vi "FTW-Tag-Core_Process.vi"(0 "FTW Actor Instance Configuration":string="{\n  \"Identity\": \"ActorName\",\n  \"InboxAddress\": \"inproc://*\",\n  \"LoggerAddress\": \"\",\n  \"My Data\": false,\n  \"Publisher URI\": \"inproc://*\",\n  \"Subscriber URIs\": \"\",\n  \"Refresh Period\": 2\n}", 11 "ErrorIn":errorcluster) -> (15 "Error":errorcluster)   [LabVIEW 2015, in "FTW-Tag-Core.lvclass"]
uses:
  FTW-Tag-Core.lvclass
  FTW-Tag-Core.lvclass/FTW-Tag-Core.ctl
  JSON/FTW-JSON-JoinMode.ctl
  Instance/FTW-ActorInstance.lvclass/FTW-ActorInstance.ctl
  JobSequencer/FTW-SEQ-Current.vi
  Message/Base/FTW-Message.lvclass
  Instance/FTW-ActorInstance.lvclass
  Message/Request/FTW-Message-IncomingRequest.lvclass
  container/FTW-Container.lvclass
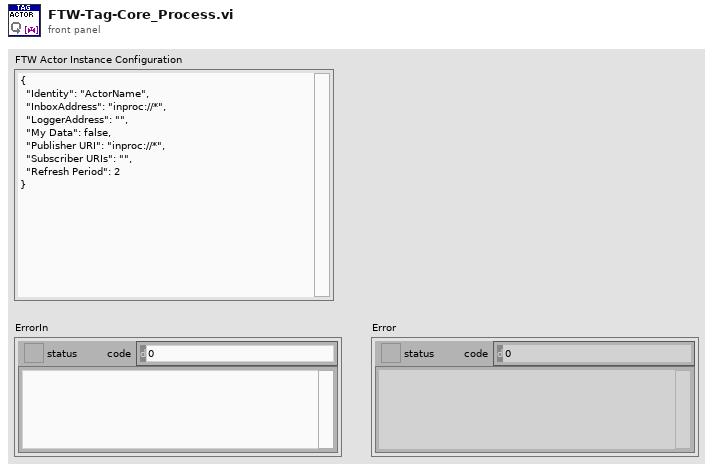
[diagram p1: front panel]
types:
  T1 = cluster{"Incoming Requests":refnum<event-registration>, "Local Messages":refnum<event-registration>, "Subscriber Registration":refnum<event-registration>}
  T2 = typedef "FTW-JSON-JoinMode.ctl" = enum32{"Upsert", "Update Only", "Insert Only"}
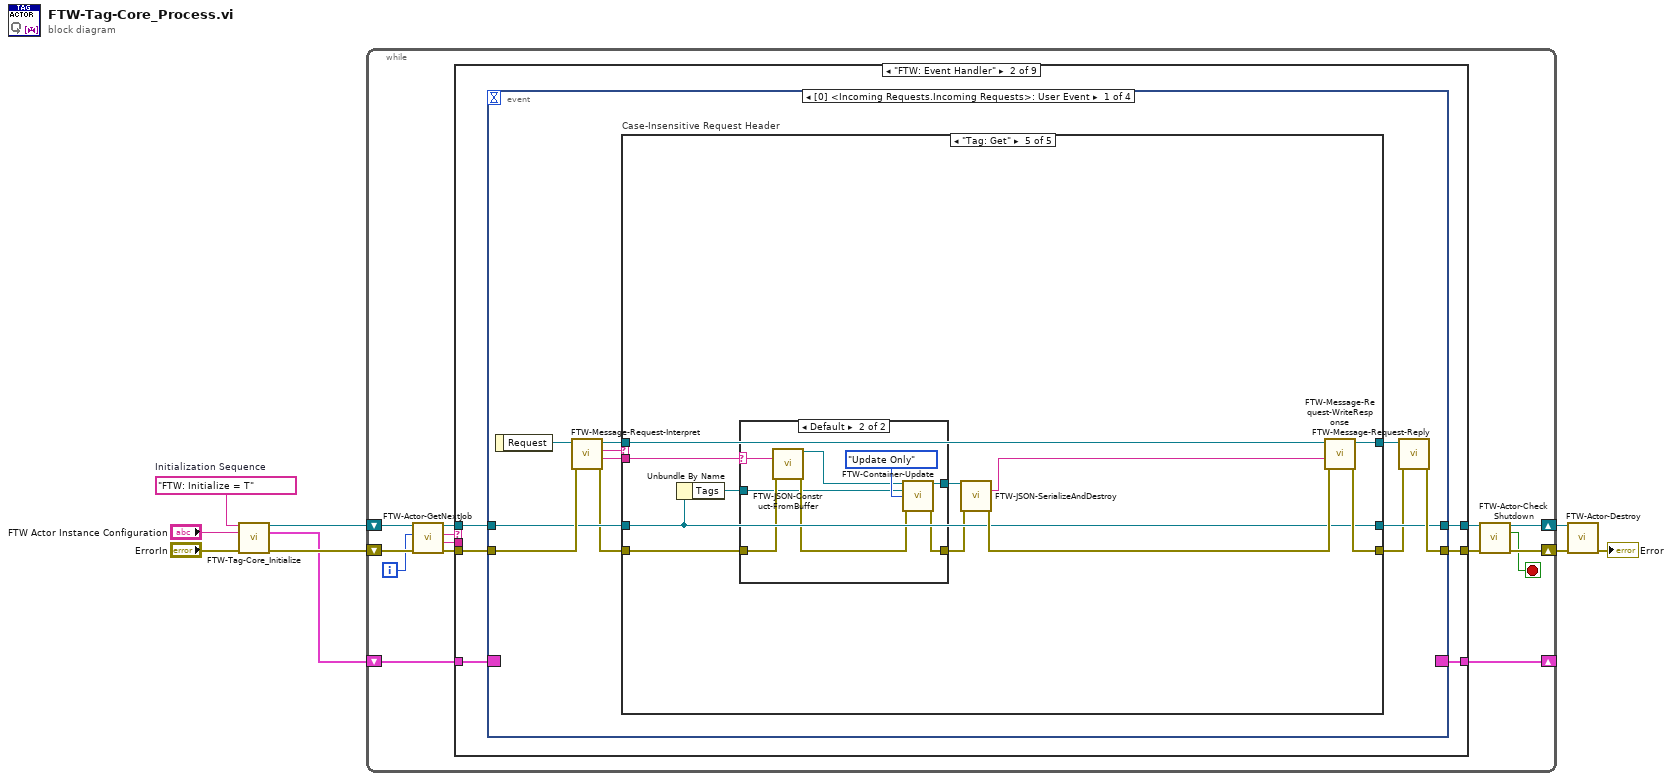
[diagram p0: block diagram]
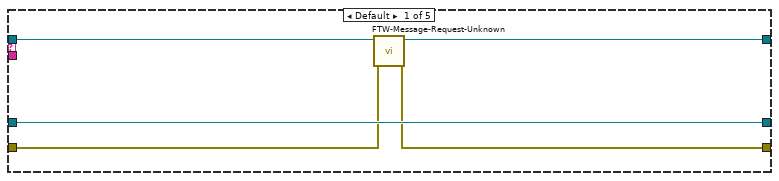
[diagram p3: hidden frame]
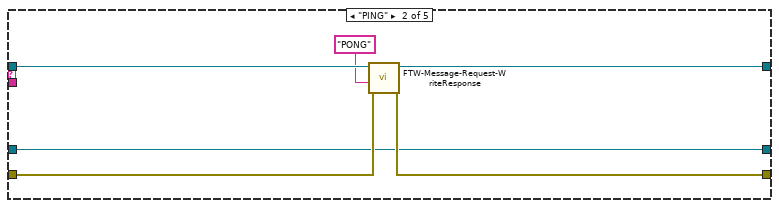
[diagram p4: hidden frame]
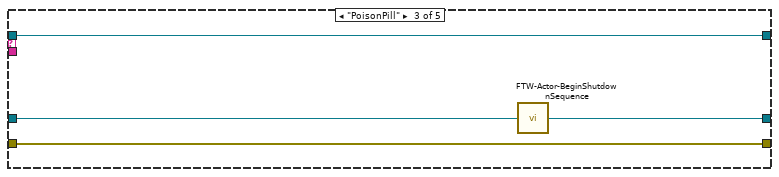
[diagram p5: hidden frame]
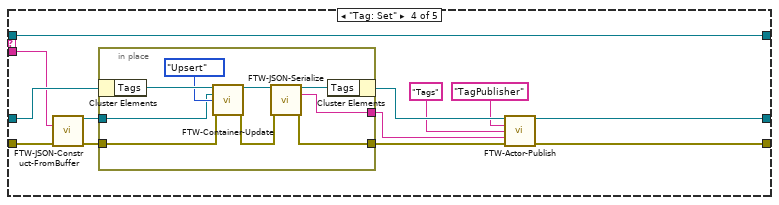
[diagram p6: hidden frame]
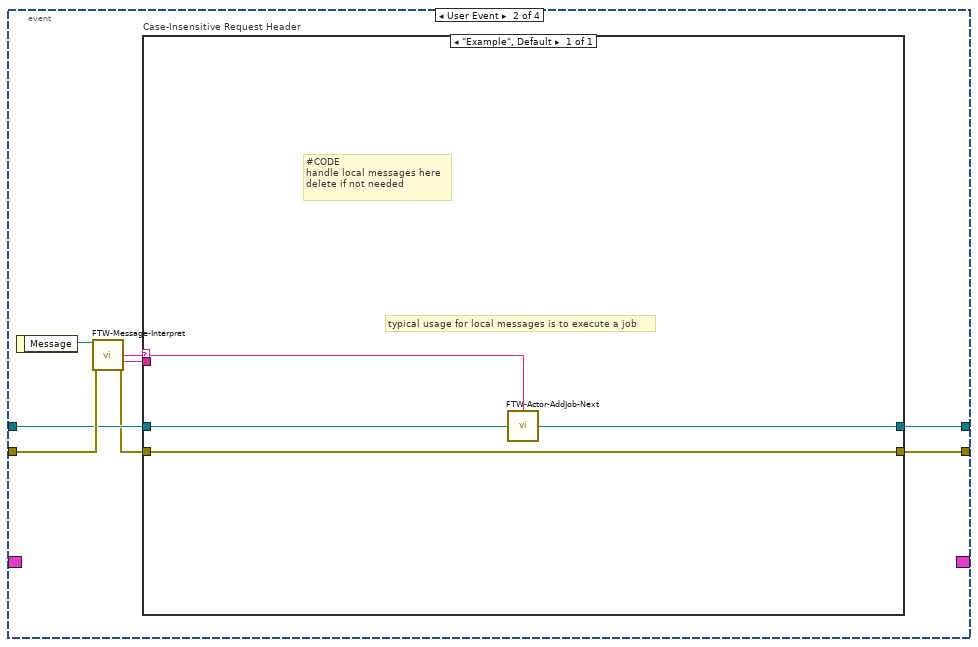
[diagram p8: hidden frame]
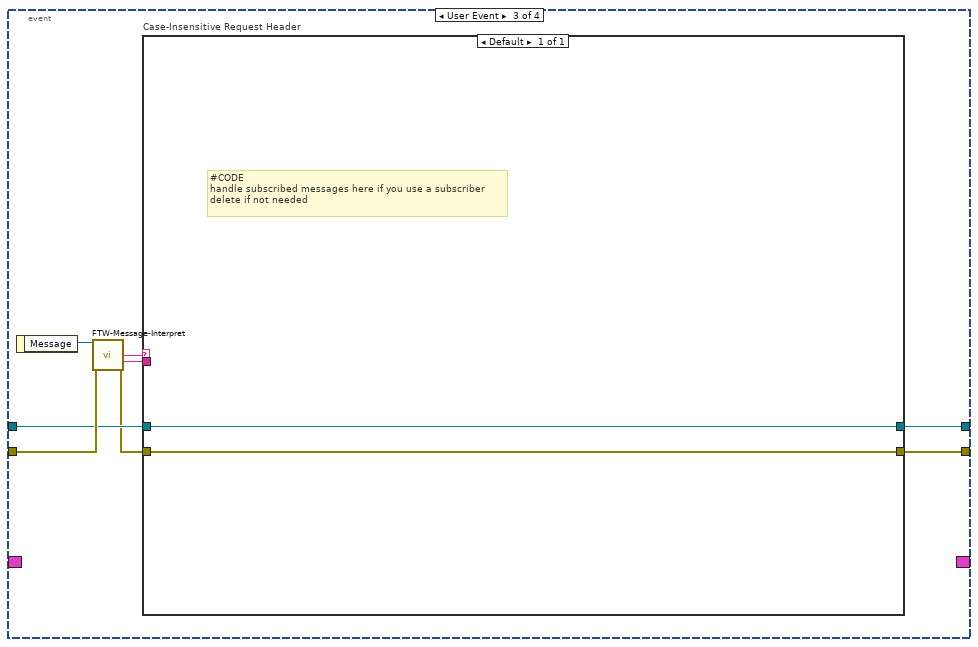
[diagram p9: hidden frame]
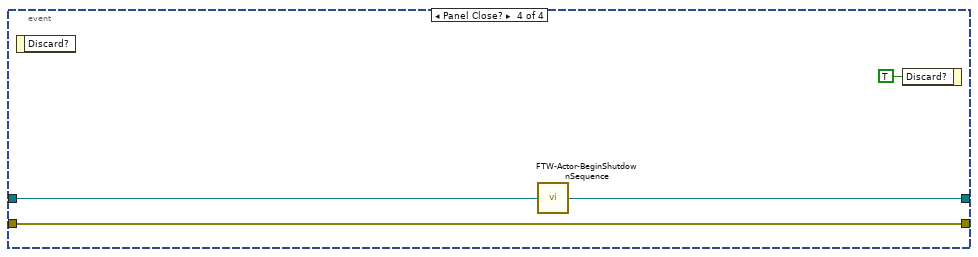
[diagram p10: hidden frame]
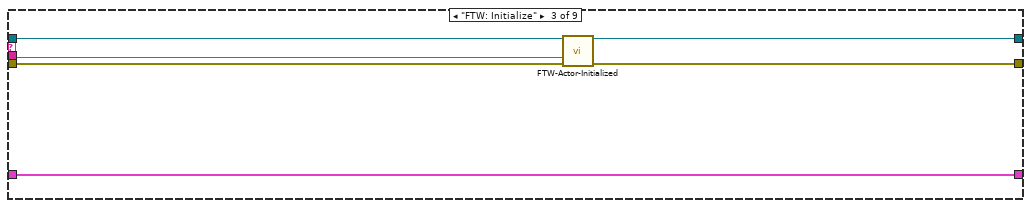
[diagram p11: hidden frame]
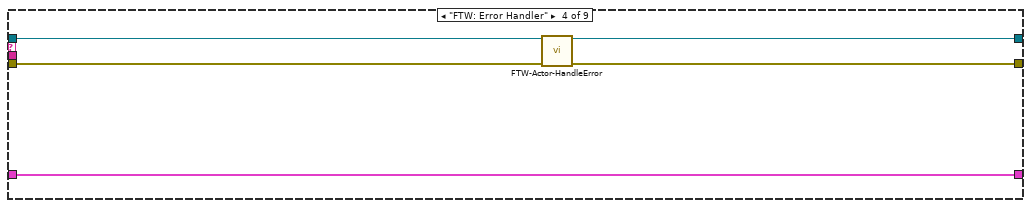
[diagram p12: hidden frame]
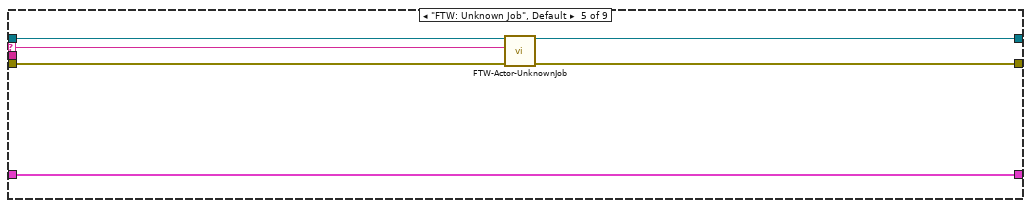
[diagram p13: hidden frame]
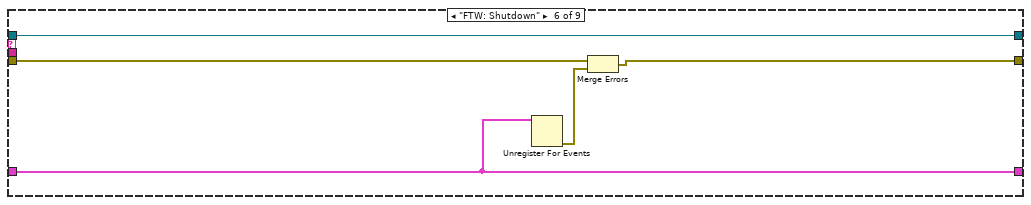
[diagram p14: hidden frame]
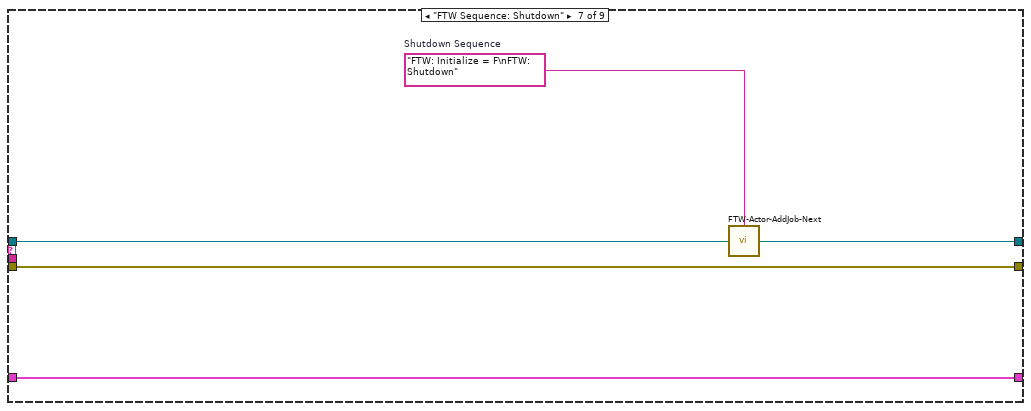
[diagram p15: hidden frame]
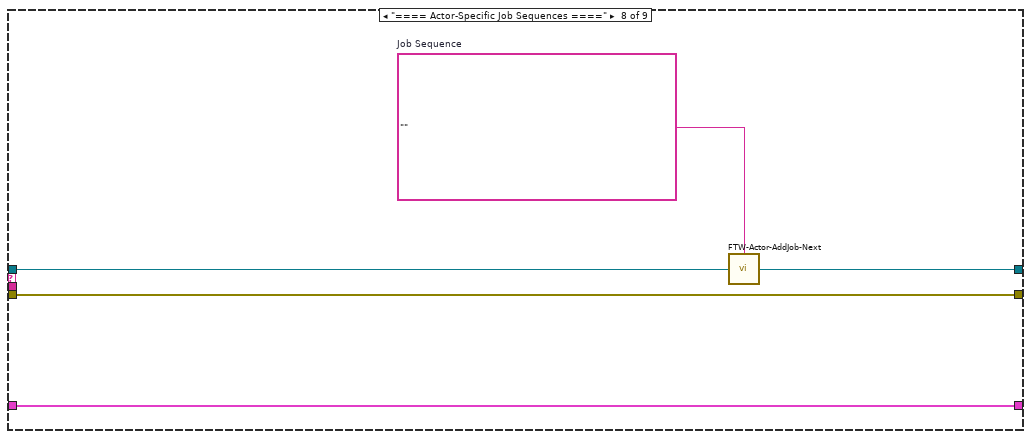
[diagram p16: hidden frame]
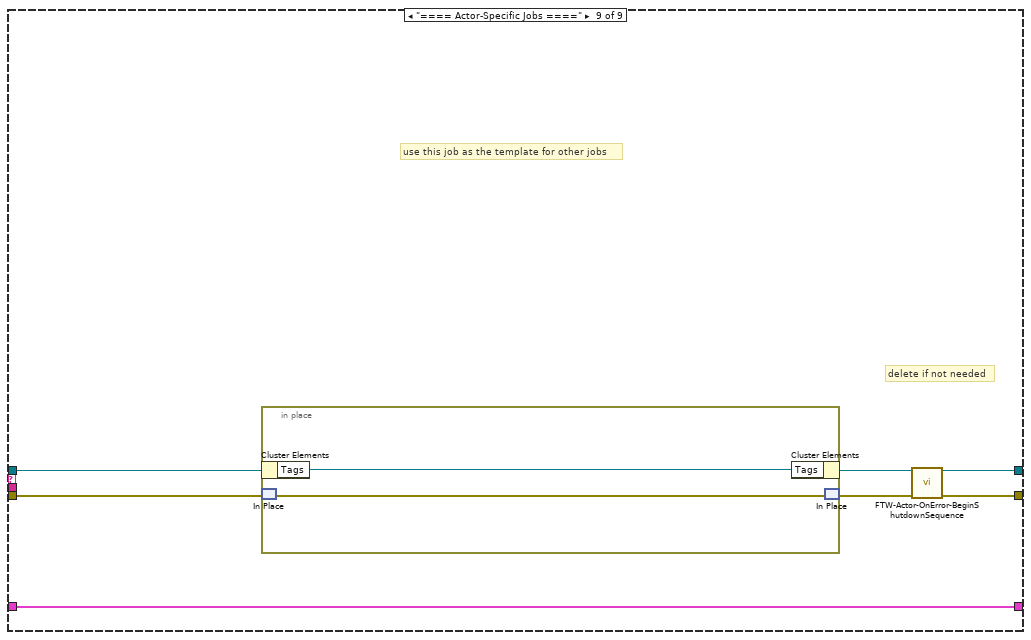
[diagram p17: hidden frame]
diagram:
  w5 = "FTW: Initialize = T"  # Initialization Sequence
  n1 = call "FTW-Tag-Core_Initialize.vi"("Initialization Sequence"=w5, "FTW Actor Instance Configuration"="FTW Actor Instance Configuration", "error in (no error)"="ErrorIn") -> ("FTW-Tag-Core Out"=w1:refnum<class "FTW-Tag-Core.lvclass">, "Event Refnums"=w2:T1, "error out"=w6:errorcluster)  [unwired: 10 in]
  n2 = while {
    shift-right: [w13] -> w8
    shift-left: w6 -> [w20]
    shift-right: [w10] -> _
    shift-left: w2 -> [w23]
    shift-right: [w15] -> w9
    shift-left: w1 -> [w22]
    i -> [w11]
    stop <- w12 stop-if-true
    n3 = call "FTW-Actor-GetNextJob.vi"("error in"=w20, "Jobs Performed"=w11, "FTW Actor Instance"=w22) -> ("error out"=w19:errorcluster, "Job Data"=w17:string, "Job Name"=w18:string, "FTW Actor Instance out"=w21:refnum<class "FTW-Tag-Core.lvclass">)  [unwired: 5 in]
    n4 = case shown="\"FTW: Event Handler\"" w18 {
      selector: w18 -> [_ _ _ _ w139 _ _ _ _]
      tunnel: [w25 w32 w130 w134 w142 w148 w153 w158 w162] -> w14
      tunnel: w19 -> [w25 w31 w133 w136 w143 w149 w153 w158 w165]
      tunnel: w23 -> [w26 w27 w132 w138 w144 w146 w154 w159 w166]
      tunnel: [w26 w30 w132 w138 w144 w146 w154 w159 w166] -> w10
      tunnel: w17 -> [_ _ w128 _ _ _ _ _ _]
      tunnel: [w24 w29 w131 w135 w140 w145 w151 w156 w160] -> w16
      tunnel: w21 -> [w24 w28 w129 w137 w141 w145 w152 w157 w163]
      frame "==== Featherweight Framework Jobs ====" {
      }
      frame "FTW: Event Handler" {
        n5 = event shown="[0] <Incoming Requests.Incoming Requests>: User Event" {
          selector: w27 -> [_ _ _ _]
          dyn-events: [_ _ _ _] -> w30
          timeout: _ -> [_ _ _ _]
          tunnel: [w42 w104 w116 w126] -> w32
          tunnel: w31 -> [w41 w108 w120 w126]
          tunnel: [w36 w105 w117 w124] -> w29
          tunnel: w28 -> [w40 w107 w119 w125]
          event User Event {
            n6 = event-data() -> ("Request"=w43:refnum<class "FTW-Message-IncomingRequest.lvclass">)  [unwired: 1 in]
            n7 = call "FTW-Message-Request-Interpret.vi"("error in"=w41, "FTW Incoming Request"=w43) -> ("error out"=w39:errorcluster, "Request Body"=w33:string, "Request Header"=w37:string, "FTW Incoming Request out"=w38:refnum<class "FTW-Message-IncomingRequest.lvclass">)  [unwired: 6 in]
            n8 = case "Case-Insensitive Request Header" shown="\"Tag: Get\"" w37 {
              tunnel: [w46 w52 w57 w64 w91] -> w35
              tunnel: w39 -> [w47 w53 w57 w70 w88]
              tunnel: [w48 w51 w58 w62 w86] -> w36
              tunnel: w40 -> [w48 w51 w56 w68 w86]
              tunnel: w38 -> [w45 w54 w55 w71 w89]
              tunnel: [w44 w50 w55 w71 w90] -> w34
              tunnel: w33 -> [_ _ _ w66 w85]
              frame Default {
                n9 = call "FTW-Message-Request-Unknown.vi"("error in"=w47, "FTW Incoming Request"=w45) -> ("error out"=w46:errorcluster, "FTW Incoming Request Out"=w44:refnum<class "FTW-Message-IncomingRequest.lvclass">)  [unwired: 8 in]
              }
              frame "PING" {
                n10 = call "FTW-Message-Request-WriteResponse.vi"("error in"=w53, "Response Body"="PONG" ("Response Header"), "FTW Incoming Request"=w54) -> ("error out"=w52:errorcluster, "FTW Incoming Request out"=w50:refnum<class "FTW-Message-IncomingRequest.lvclass">)  [unwired: 7 in]
              }
              frame "PoisonPill" {
                n11 = call "FTW-Actor-BeginShutdownSequence.vi"("FTW Actor Instance"=w56) -> ("FTW Actor Instance out"=w58:refnum<class "FTW-Tag-Core.lvclass">)  [unwired: 3 in]
              }
              frame "Tag: Set" {
                n12 = call "FTW-JSON-Construct-FromBuffer.vi"("JSON String (UTF-8)"=w66, "error in"=w70) -> ("JSON"=w65:refnum<class "FTW-Container.lvclass">, "error out"=w67:errorcluster)  [unwired: 12 in]
                n13 = in-place {
                  in-place-border: w67 -> [w80]
                  in-place-border: [w78] -> w69
                  in-place-border: [w74] -> w59
                  in-place-border: w65 -> [w72]
                  n14 = in-place-cluster #1(w68) -> ("Tags"=w76:refnum<class "FTW-Container.lvclass">)
                  n15 = call "FTW-Container-Update.vi"("FTW-Container In"=w76, "Other Container"=w72, "Join Mode"=FTW-JSON-JoinMode."Upsert", "error in"=w80) -> ("Updated Container"=w77:refnum<class "FTW-Container.lvclass">, "error out"=w79:errorcluster)  [unwired: 10 in]
                  n16 = call "FTW-JSON-Serialize.vi"("JSON"=w77, "error in"=w79) -> ("JSON out"=w75:refnum<class "FTW-Container.lvclass">, "JSON String (UTF-8)"=w74:string, "error out"=w78:errorcluster)  [unwired: 11 in]
                  n17 = in-place-cluster #1("Tags"=w75) -> (w63:refnum<class "FTW-Tag-Core.lvclass">)
                }
                n18 = call "FTW-Actor-Publish.vi"("FTW-ActorExtended In"=w63, "Publisher Name"="TagPublisher", "Message Header"="Tags", "Message Body"=w59, "error in"=w69) -> ("FTW-ActorExtended Out"=w62:refnum<class "FTW-Tag-Core.lvclass">, "error out"=w64:errorcluster)  [unwired: 9 in]
              }
              frame "Tag: Get" {
                n19 = Unbundle By Name(w86) -> ("Tags"=w81:refnum<class "FTW-Container.lvclass">)
                n20 = case shown="Default" w85 {
                  selector: w85 -> [_ w99]
                  tunnel: w88 -> [w92 w101]
                  tunnel: [w92 w98] -> w83
                  tunnel: [w93 w97] -> w82
                  tunnel: w81 -> [w93 w95]
                  frame "\u0000" {
                  }
                  frame Default {
                    n21 = call "FTW-JSON-Construct-FromBuffer.vi"("JSON String (UTF-8)"=w99, "error in"=w101) -> ("JSON"=w94:refnum<class "FTW-Container.lvclass">, "error out"=w100:errorcluster)  [unwired: 12 in]
                    n22 = call "FTW-Container-Update.vi"("FTW-Container In"=w94, "Other Container"=w95, "Join Mode"=FTW-JSON-JoinMode."Update Only", "error in"=w100) -> ("Updated Container"=w97:refnum<class "FTW-Container.lvclass">, "error out"=w98:errorcluster)  [unwired: 10 in]
                  }
                }
                n23 = call "FTW-JSON-SerializeAndDestroy.vi"("JSON"=w82, "error in"=w83) -> ("JSON String (UTF-8)"=w84:string, "error out"=w87:errorcluster)  [unwired: 12 in]
                n24 = call "FTW-Message-Request-WriteResponse.vi"("error in"=w87, "Response Body"=w84, "FTW Incoming Request"=w89) -> ("error out"=w91:errorcluster, "FTW Incoming Request out"=w90:refnum<class "FTW-Message-IncomingRequest.lvclass">)  [unwired: 7 in]
              }
            }
            n25 = call "FTW-Message-Request-Reply.vi"("FTW: Reply Error"=w35, "FTW Incoming Request"=w34) -> ("error out"=w42:errorcluster)  [unwired: 8 in, 1 out]
          }
          event User Event {
            n26 = event-data() -> ("Message"=w109:refnum<class "FTW-Message.lvclass">)  [unwired: 1 in]
            n27 = call-dynamic "FTW-Message-Interpret.vi"("FTW Message"=w109, "error in"=w108) -> ("Message Header"=w103:string, "Message Body"=w102:string, "error out"=w106:errorcluster)  [unwired: 9 in, 2 out]
            n28 = case "Case-Insensitive Request Header" shown="\"Example\", Default" w103 {
              selector: w103 -> [w110]
              tunnel: [w112] -> w104
              tunnel: w106 -> [w112]
              tunnel: [w111] -> w105
              tunnel: w107 -> [w113]
              tunnel: w102 -> [_]
              frame "Example", Default {
                # "#CODE\nhandle local messages here\ndelete if not needed"
                # "typical usage for local messages is to execute a job"
                n29 = call "FTW-Actor-AddJob-Next.vi"("Add Next in Job Queue"=w110, "FTW Actor Instance"=w113) -> ("FTW Actor Instance out"=w111:refnum<class "FTW-Tag-Core.lvclass">)  [unwired: 2 in]
              }
            }
          }
          event User Event {
            n30 = event-data() -> ("Message"=w121:refnum<class "FTW-Message.lvclass">)  [unwired: 1 in]
            n31 = call-dynamic "FTW-Message-Interpret.vi"("FTW Message"=w121, "error in"=w120) -> ("Message Header"=w115:string, "Message Body"=w114:string, "error out"=w118:errorcluster)  [unwired: 9 in, 2 out]
            n32 = case "Case-Insensitive Request Header" shown="Default" w115 {
              tunnel: [w122] -> w116
              tunnel: w118 -> [w122]
              tunnel: [w123] -> w117
              tunnel: w119 -> [w123]
              tunnel: w114 -> [_]
              frame Default {
                # "#CODE\nhandle subscribed messages here if you use a subscriber\ndelete if not needed"
              }
            }
          }
          event Panel Close? {
            n33 = event-data() -> ()  [unwired: 1 in, 1 out]
            n34 = call "FTW-Actor-BeginShutdownSequence.vi"("FTW Actor Instance"=w125) -> ("FTW Actor Instance out"=w124:refnum<class "FTW-Tag-Core.lvclass">)  [unwired: 3 in]
            n35 = event-data("Discard?"=TRUE) -> ()  [unwired: 1 in, 1 out]
          }
        }
      }
      frame "FTW: Initialize" {
        n36 = call-dynamic "FTW-Actor-Initialized.vi"("FTW Actor Instance"=w129, "Positive Init?"=w128, "error in"=w133) -> ("FTW Actor Instance out"=w131:refnum<class "FTW-Tag-Core.lvclass">, "error out"=w130:errorcluster)  [unwired: 11 in]
      }
      frame "FTW: Error Handler" {
        n37 = call-dynamic "FTW-Actor-HandleError.vi"("FTW Actor Instance"=w137, "error in"=w136) -> ("FTW Actor Instance out"=w135:refnum<class "FTW-Tag-Core.lvclass">, "error out"=w134:errorcluster)  [unwired: 10 in, 2 out]
      }
      frame "FTW: Unknown Job", Default {
        n38 = call-dynamic "FTW-Actor-UnknownJob.vi"("FTW Actor Instance"=w141, "Unknown Job"=w139, "error in"=w143) -> ("FTW Actor Instance out"=w140:refnum<class "FTW-Tag-Core.lvclass">, "error out"=w142:errorcluster)  [unwired: 11 in]
      }
      frame "FTW: Shutdown" {
        n39 = Unregister For Events(event registration refnum=w146) -> (error out=w147:errorcluster)  [unwired: 1 in]
        n40 = Merge Errors(w149, w147) -> (w148:errorcluster)
      }
      frame "FTW Sequence: Shutdown" {
        w150 = "FTW: Initialize = F\nFTW: Shutdown"  # Shutdown Sequence
        n41 = call "FTW-Actor-AddJob-Next.vi"("Add Next in Job Queue"=w150, "FTW Actor Instance"=w152) -> ("FTW Actor Instance out"=w151:refnum<class "FTW-Tag-Core.lvclass">)  [unwired: 2 in]
      }
      frame "==== Actor-Specific Job Sequences ====" {
        w155 = ""  # Job Sequence
        n42 = call "FTW-Actor-AddJob-Next.vi"("Add Next in Job Queue"=w155, "FTW Actor Instance"=w157) -> ("FTW Actor Instance out"=w156:refnum<class "FTW-Tag-Core.lvclass">)  [unwired: 2 in]
      }
      frame "==== Actor-Specific Jobs ====" {
        # "delete if not needed"
        # "use this job as the template for other jobs"
        n43 = in-place {
          n44 = in-place-cluster #2(w163) -> ("Tags"=w167:refnum<class "FTW-Container.lvclass">)
          n45 = in-place-match #3(w165) -> (w168:errorcluster)
          n46 = in-place-cluster #2("Tags"=w167) -> (w161:refnum<class "FTW-Tag-Core.lvclass">)
          n47 = in-place-match #3(w168) -> (w164:errorcluster)
        }
        n48 = call-dynamic "FTW-Actor-OnError-BeginShutdownSequence.vi"("FTW Actor Instance"=w161, "error in"=w164) -> ("FTW Actor Instance out"=w160:refnum<class "FTW-Tag-Core.lvclass">, "error out"=w162:errorcluster)  [unwired: 12 in]
      }
    }
    n49 = call "FTW-Actor-CheckShutdown.vi"("FTW Actor Instance"=w16, "error in"=w14) -> ("FTW Actor Instance out"=w15:refnum<class "FTW-Tag-Core.lvclass">, "Shutdown?"=w12:bool, "error out"=w13:errorcluster)  [unwired: 11 in]
  }
  n50 = call-dynamic "FTW-Actor-Destroy.vi"("FTW Actor Instance"=w9, "error in"=w8) -> ("error out"=→"Error":errorcluster)  [unwired: 13 in]
